vi "Transform.vi"(8 "error in (no error)":errorcluster caption="entrée d'erreur (pas d'erreur)", 9 "y":string[][](array[string]), 10 "X":string[][](array[string]), 11 "SkewedChi2Sampler.lvclass":refnum<class "SkewedChi2Sampler.lvclass">) -> (0 "error in (no error)":errorcluster caption="entrée d'erreur (pas d'erreur)", 2 "Data":T1, 3 "SkewedChi2Sampler.lvclass":refnum<class "SkewedChi2Sampler.lvclass">)   [LabVIEW 2020, in "SkewedChi2Sampler.lvclass"]
doc: "Apply the approximate feature map to X.\n\nReturns : \n\n- X_new : array-like, shape (n_samples, n_components)"
uses:
  SkewedChi2Sampler.lvclass
  SkewedChi2Sampler.lvclass/SkewedChi2Sampler.ctl
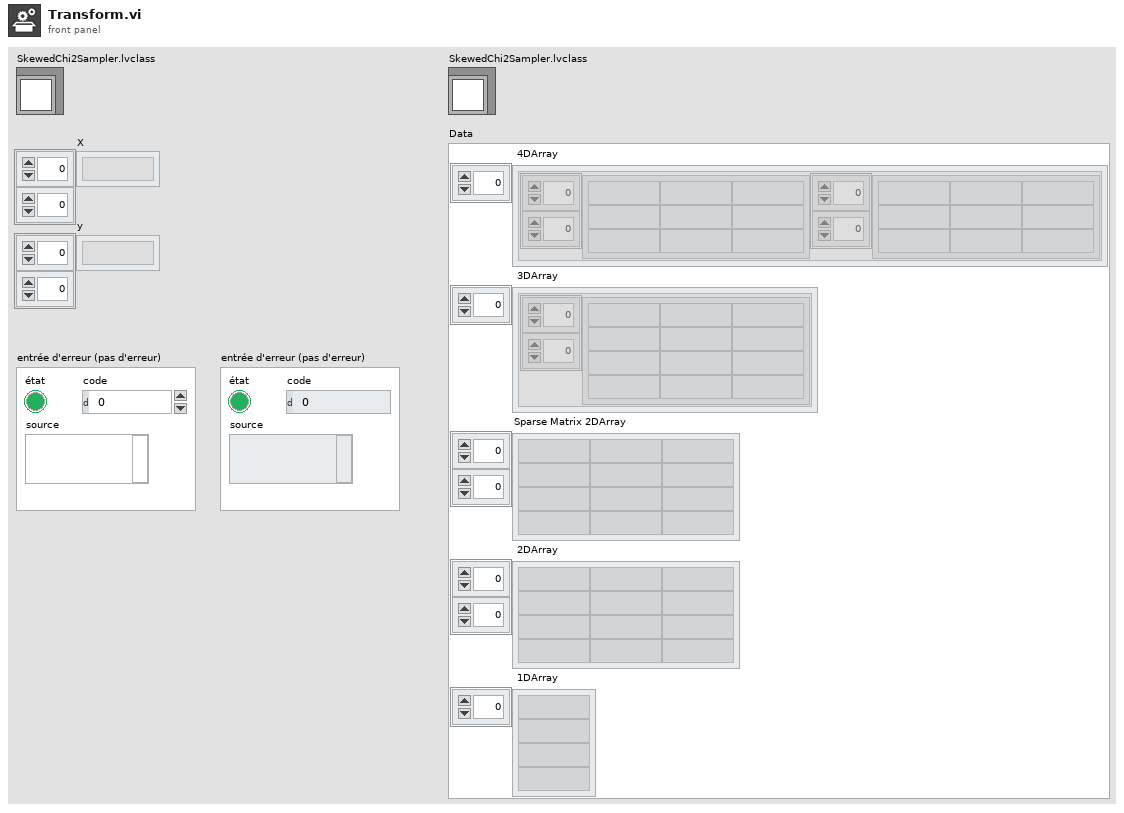
[diagram p1: front panel]
types:
  T1 = cluster{" 4DArray":cluster{"1":string[][], "2":string[][]}[], " 3DArray":cluster{"Tableau":string[][]}[], "Sparse Matrix 2DArray":string[][], " 2DArray":string[][], " 1DArray":string[]}
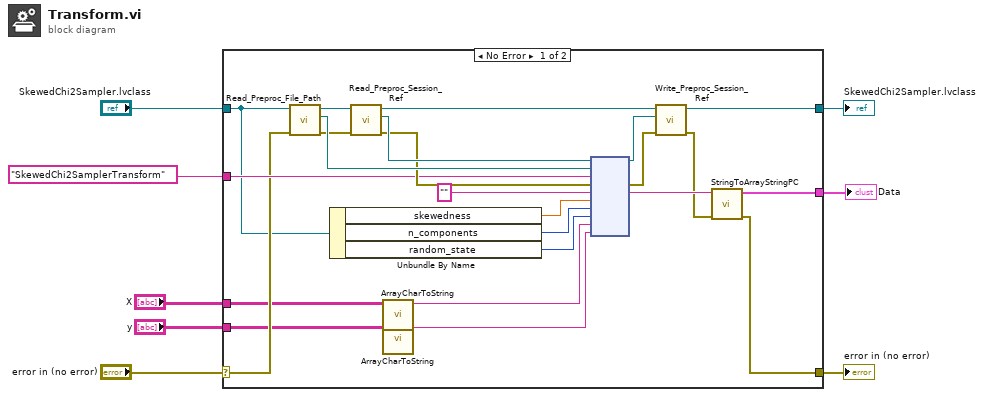
[diagram p0: block diagram]
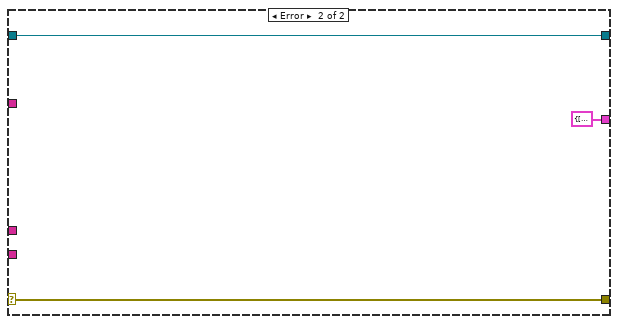
[diagram p2: hidden frame]
diagram:
  n1 = case shown="No Error" "error in (no error)" {
    selector: "error in (no error)" -> [w20 w35]
    tunnel: [w14 w35] -> w7
    tunnel: [w17 w34] -> w5
    tunnel: "SkewedChi2Sampler.lvclass" -> [w19 w34]
    tunnel: "SkewedChi2SamplerTransform" ("Fonction") -> [w21 _]
    tunnel: "X" -> [w12 _]
    tunnel: [w13 T1 {" 4DArray"=[], " 3DArray"=[], "Sparse Matrix 2DArray"=[], " 2DArray"=[], " 1DArray"=[]} ("Data")] -> w1
    tunnel: "y" -> [w10 _]
    frame No Error {
      n2 = call-dynamic "Read_Preproc_File_Path.vi"("error in (no error)"=w20, "Python in"=w19) -> ("error out"=w27:errorcluster, "File_Path"=w30:path, "Python out"=w32:refnum<class "SkewedChi2Sampler.lvclass">)  [unwired: 7 in]
      n3 = Unbundle By Name(w19) -> ("skewedness"=w23:dbl, "n_components"=w22:i32, "random_state"=w18:i32)
      n4 = call-dynamic "Read_Preproc_Session_Ref.vi"("error in (no error)"=w27, "Python in"=w32) -> ("error out"=w28:errorcluster, "Session_ref"=w29:refnum<k35>, "Python out"=w31:refnum<class "SkewedChi2Sampler.lvclass">)  [unwired: 7 in]
      n5 = call "ArrayCharToString.vi"("TAB"=w12) -> ("Instruction"=w11:string)  [unwired: 10 in]
      n6 = call "ArrayCharToString.vi"("TAB"=w10) -> ("Instruction"=w9:string)  [unwired: 10 in]
      n7 = node(w29, w30, w21, w28, "", w23, w22, w18, w11, w9) -> (w24:refnum<k35>, w26:errorcluster, w16:string)  [unwired: 5 in, 2 out]
      n8 = call-dynamic "Write_Preproc_Session_Ref.vi"("error in (no error)"=w26, "Session_ref"=w24, "Python in"=w31) -> ("error out"=w15:errorcluster, "Python out"=w17:refnum<class "SkewedChi2Sampler.lvclass">)  [unwired: 7 in]
      n9 = call "StringToArrayStringPC.vi"("sortie d'erreur"=w15, "Return value"=w16) -> ("sortie d'erreur"=w14:errorcluster, "Data"=w13:T1)  [unwired: 8 in]
    }
    frame Error {
    }
  }
  "error in (no error)" <- w7
  "SkewedChi2Sampler.lvclass" <- w5
  "Data" <- w1
